vi "normalize-vec.vi"(11 "Vec Input":dbl[](array[numeric])) -> (0 "index2":dbl, 1 "index1":dbl, 2 "index0":dbl, 3 "Array Output":dbl[](array[numeric]))   [LabVIEW 2017]
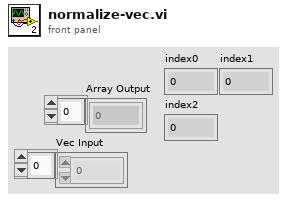
[diagram p1: front panel]
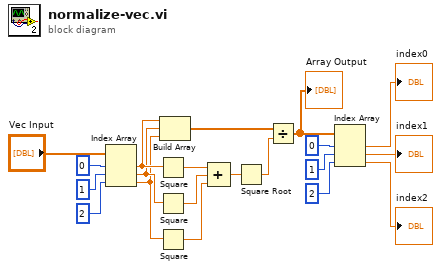
[diagram p0: block diagram]
diagram:
  n1 = Index Array(array="Vec Input", index #1=0 ("index"), index #2=1 ("index"), index #3=2 ("index")) -> (element #1=w5:dbl, element #2=w4:dbl, element #3=w3:dbl)
  n2 = Square(x=w5) -> (x^2=w17:dbl)
  n3 = Square(x=w4) -> (x^2=w18:dbl)
  n4 = Square(x=w3) -> (x^2=w19:dbl)
  n5 = Build Array(w5, w4, w3) -> (w20:dbl[])
  n6 = Compound Arithmetic op=ADD(w17, w18, w19) -> (w2:dbl)
  n7 = Square Root(x=w2) -> (sqrt(x)=w1:dbl)
  n8 = Divide(x=w20, y=w1) -> (x/y=w16:dbl[])
  "Array Output" <- w16
  n9 = Index Array(array=w16, index #1=0 ("index"), index #2=1 ("index"), index #3=2 ("index")) -> (element #1=→"index0":dbl, element #2=→"index1":dbl, element #3=→"index2":dbl)
